vi "Remove Device.vi"(8 "error in (no error)":errorcluster, 10 "Device":refnum<class "Hardware.lvclass">, 11 "Controller in":refnum<class "Controller.lvclass">) -> (0 "error out":errorcluster, 3 "Controller out":refnum<class "Controller.lvclass">)   [LabVIEW 2016, in "Controller Actor.lvlib" / "Controller.lvclass"]
uses:
  <userlib>/Common Components/Controller/Controller.lvclass
  C:/Program Files (x86)/National Instruments/LabVIEW 2016/vi.lib/ActorFramework/Actor/Actor.lvclass
  <userlib>/Common Components/Hardware/Abstract Hardware/Hardware.lvclass
  <userlib>/Common Components/Controller/Controller.lvclass/Controller.ctl
  <vilib>/ActorFramework/Actor/Actor.lvclass/Actor.ctl
  <vilib>/ActorFramework/Message Enqueuer/Message Enqueuer.lvclass/Message Enqueuer.ctl
  <vilib>/ActorFramework/Message Enqueuer/Init from Existing Queue.vi
  <vilib>/ActorFramework/Message Enqueuer/Message Enqueuer.lvclass
  <userlib>/Common Components/Controller/Messages/Log Status/Log Status.lvclass
  <vilib>/ActorFramework/Actor/Actor.lvclass
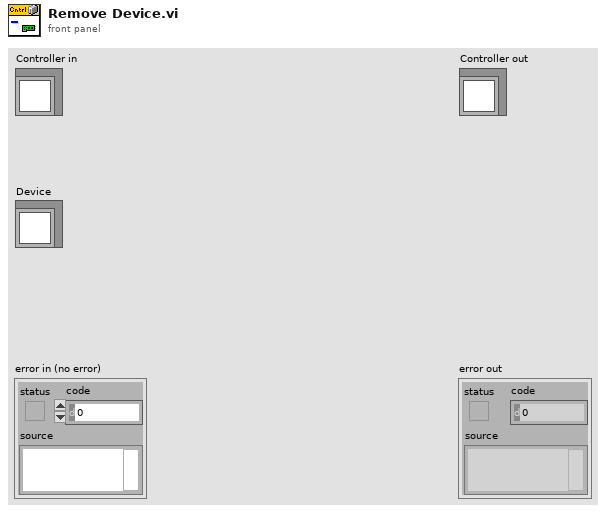
[diagram p1: front panel]
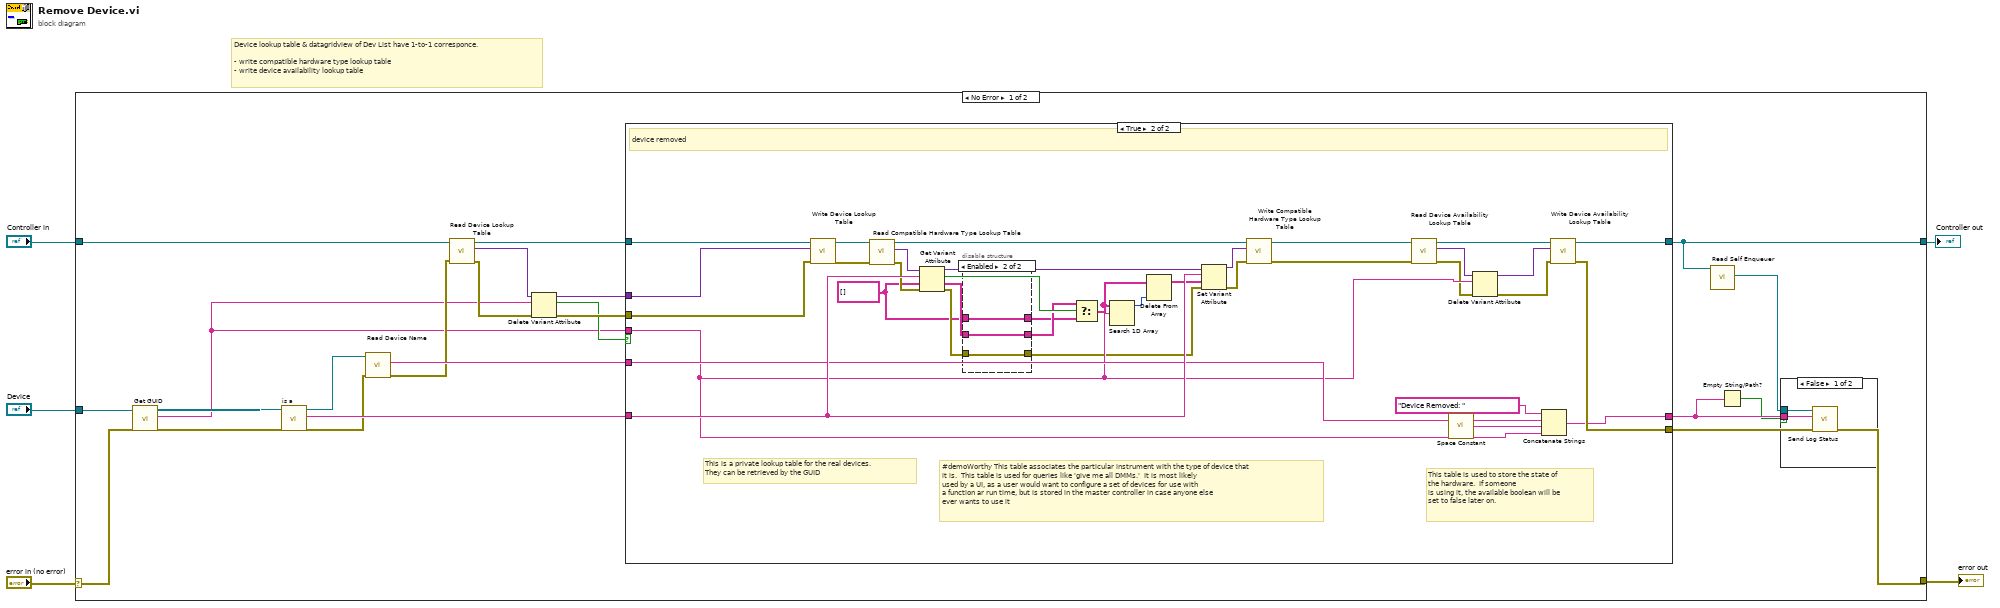
[diagram p0: block diagram]
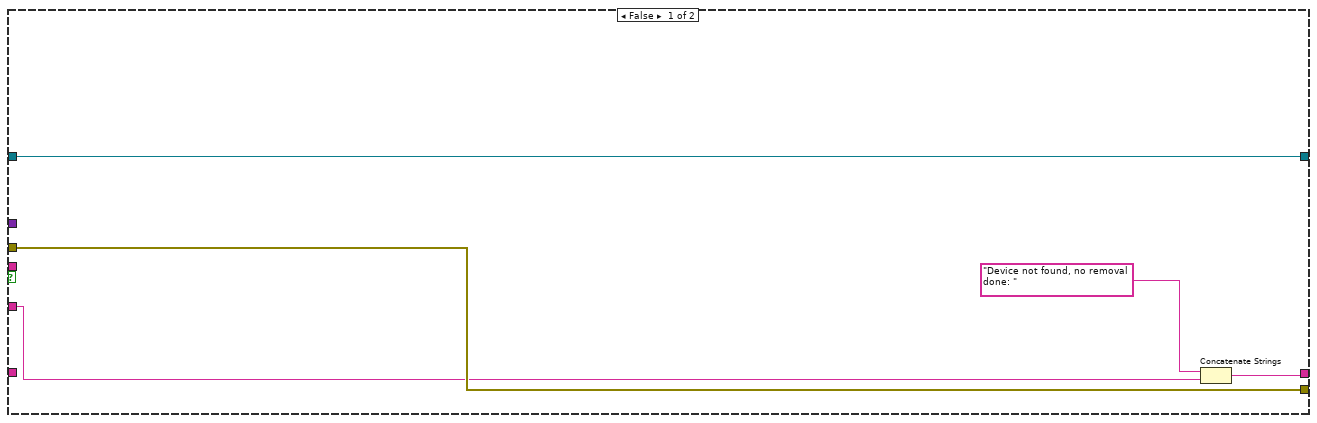
[diagram p3: hidden frame]
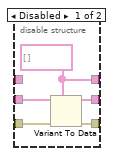
[diagram p4: hidden frame]
diagram:
  # "Device lookup table & datagridview of Dev List have 1-to-1 corresponce.\n\n- write compatible hardware type lookup table\n- write device availability lookup table"
  n1 = case shown="No Error" "error in (no error)" {
    selector: "error in (no error)" -> [w8 w80]
    tunnel: [w26 w80] -> w4
    tunnel: [w19 w79] -> w2
    tunnel: "Controller in" -> [w14 w79]
    tunnel: "Device" -> [w15 _]
    frame No Error {
      n2 = call <userlib>:"Get GUID.vi"("error in (no error)"=w8, "Hardware in"=w15) -> ("error out"=w7:errorcluster, "GUID"=w6:string, "Hardware out"=w9:refnum<class "Hardware.lvclass">)  [unwired: 7 in]
      n3 = call-dynamic "is a.vi"("error in (no error)"=w7, "Hardware in"=w9) -> ("error out"=w24:errorcluster, "is a"=w27:string, "Hardware out"=w25:refnum<class "Hardware.lvclass">)  [unwired: 7 in]
      n4 = call <userlib>:"Read Device Name.vi"("error in (no error)"=w24, "Analog in"=w25) -> ("error out"=w10:errorcluster, "Device Name"=w22:string)  [unwired: 7 in, 1 out]
      n5 = call <userlib>:"Read Device Lookup Table.vi"("error in (no error)"=w10, "Controller in"=w14) -> ("error out"=w11:errorcluster, "Device Lookup Table (Device GUID -> Device Object)"=w12:variant, "Controller out"=w13:refnum<class "Controller.lvclass">)  [unwired: 7 in]
      n6 = Delete Variant Attribute(4:w11, 6:w6, 7:w12) -> (0:w21:errorcluster, 2:w18:bool, 3:w23:variant)
      n7 = case shown="True" w18 {
        tunnel: w27 -> [_ w70]
        tunnel: [w33 w69] -> w26
        tunnel: w13 -> [w34 w68]
        tunnel: w23 -> [_ w67]
        tunnel: w22 -> [w30 w66]
        tunnel: w21 -> [w33 w65]
        tunnel: [w34 w64] -> w19
        tunnel: [w31 w63] -> w17
        tunnel: w6 -> [_ w62]
        frame False {
          n8 = Concatenate Strings("Device not found, no removal done: " ("string"), w30) -> (w31:string)
        }
        frame True {
          w38 = string[] []
          # "This table is used to store the state of the hardware.  If someone\nis using it, the available boolean will be set to false later on."
          # "This is a private lookup table for the real devices.  \nThey can be retrieved by the GUID"
          # "#demoWorthy This table associates the particular instrument with the type of device that\nit is.  This table is used for queries like 'give me all DMMs.'  It is most likely\nused by a UI, as a user would want to configure a set of devices for use with\na function ar run time, but is stored in the master controller in case anyone else\never wants to use it"
          # "device removed"
          n9 = call <userlib>:"Write Device Lookup Table.vi"("error in (no error)"=w65, "Device Lookup Table (Device GUID -> Device Object)"=w67, "Controller in"=w68) -> ("error out"=w47:errorcluster, "Controller out"=w55:refnum<class "Controller.lvclass">)  [unwired: 7 in]
          n10 = call <userlib>:"Read Compatible Hardware Type Lookup Table.vi"("error in (no error)"=w47, "Controller in"=w55) -> ("error out"=w48:errorcluster, "Compatible Hardware Type Lookup Table"=w52:variant, "Controller out"=w54:refnum<class "Controller.lvclass">)  [unwired: 7 in]
          n11 = Get Variant Attribute(Variant=w52, name=w70, default value (empty Variant)=w38, error in=w48) -> (duplicate Variant=w56:variant, found=w59:bool, value=w61:string[], error out=w46:errorcluster)
          n12 = disable-structure shown="Enabled" {
            disable-tunnel: w61 -> [w75 w78]
            disable-tunnel: [w74 w78] -> w58
            disable-tunnel: [w73 w76] -> w57
            disable-tunnel: w46 -> [w72 w77]
            disable-tunnel: [w71 w77] -> w45
            disable-tunnel: w38 -> [_ w76]
            frame Disabled {
              w73 = string[] []
              n13 = Variant To Data(error in=w72, type=w73, Variant=w75) -> (data=w74:string[], error out=w71:errorcluster)
            }
            frame Enabled {
            }
          }
          n14 = Select(t=w58, s=w59, f=w57) -> (s? t:f=w37:string[])
          n15 = Search 1D Array(1D array=w37, element=w62) -> (index of element=w60:i32)  [unwired: 1 in]
          n16 = Delete From Array(array=w37, index=w60) -> (array with subset deleted=w36:string[])  [unwired: 1 in, 1 out]
          n17 = Set Variant Attribute(Variant=w56, name=w70, value=w36, error in=w45) -> (Variant out=w53:variant, error out=w44:errorcluster)  [unwired: 1 out]
          n18 = call <userlib>:"Write Compatible Hardware Type Lookup Table.vi"("error in (no error)"=w44, "Compatible Hardware Type Lookup Table"=w53, "Controller in"=w54) -> ("error out"=w43:errorcluster, "Controller out"=w51:refnum<class "Controller.lvclass">)  [unwired: 7 in]
          n19 = call <userlib>:"Read Device Availability Lookup Table.vi"("error in (no error)"=w43, "Controller in"=w51) -> ("error out"=w42:errorcluster, "Device Availability Lookup Table"=w35:variant, "Controller out"=w49:refnum<class "Controller.lvclass">)  [unwired: 7 in]
          n20 = call <vilib>:"Space Constant.vi"() -> ("String"=w39:string)
          n21 = Delete Variant Attribute(4:w42, 6:w62, 7:w35) -> (0:w41:errorcluster, 3:w50:variant)  [unwired: 1 out]
          n22 = Concatenate Strings("Device Removed: " ("string"), w66, w39, w62) -> (w63:string)
          n23 = call <userlib>:"Write Device Availability Lookup Table.vi"("error in (no error)"=w41, "Device Availability Lookup Table"=w50, "Controller in"=w49) -> ("error out"=w69:errorcluster, "Controller out"=w64:refnum<class "Controller.lvclass">)  [unwired: 7 in]
        }
      }
      n24 = call <vilib>:"Read Self Enqueuer.vi"("Actor"=w19) -> ("Self Enqueuer"=w20:refnum<class "Message Enqueuer.lvclass">)  [unwired: 10 in]
      n25 = Empty String/Path?(string/path=w17) -> (empty?=w16:bool)
      n26 = case shown="False" w16 {
        tunnel: w20 -> [w29 _]
        tunnel: w17 -> [w28 _]
        frame False {
          n27 = call <userlib>:"Send Log Status.vi"("String"=w28, "Message Enqueuer in"=w29) -> ()  [unwired: 8 in, 2 out]
        }
        frame True {
        }
      }
    }
    frame Error {
    }
  }
  "error out" <- w4
  "Controller out" <- w2
